vi "Grab Image from D-Link.vi"(8 "error in (no error)":errorcluster, 11 "address":string="169.254.66.10") -> (0 "error out":errorcluster, 3 "data out":string)   [LabVIEW 2012]
panel:
  out "bytes written":i32
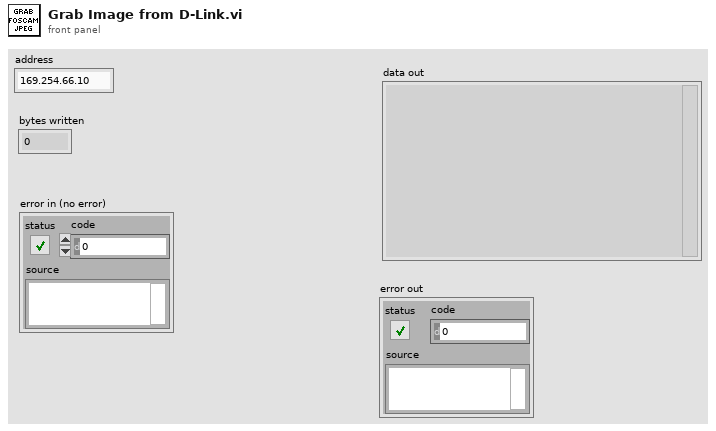
[diagram p1: front panel]
types:
  T1 = enum16{"Standard", "Buffered", "CRLF", "Immediate"}
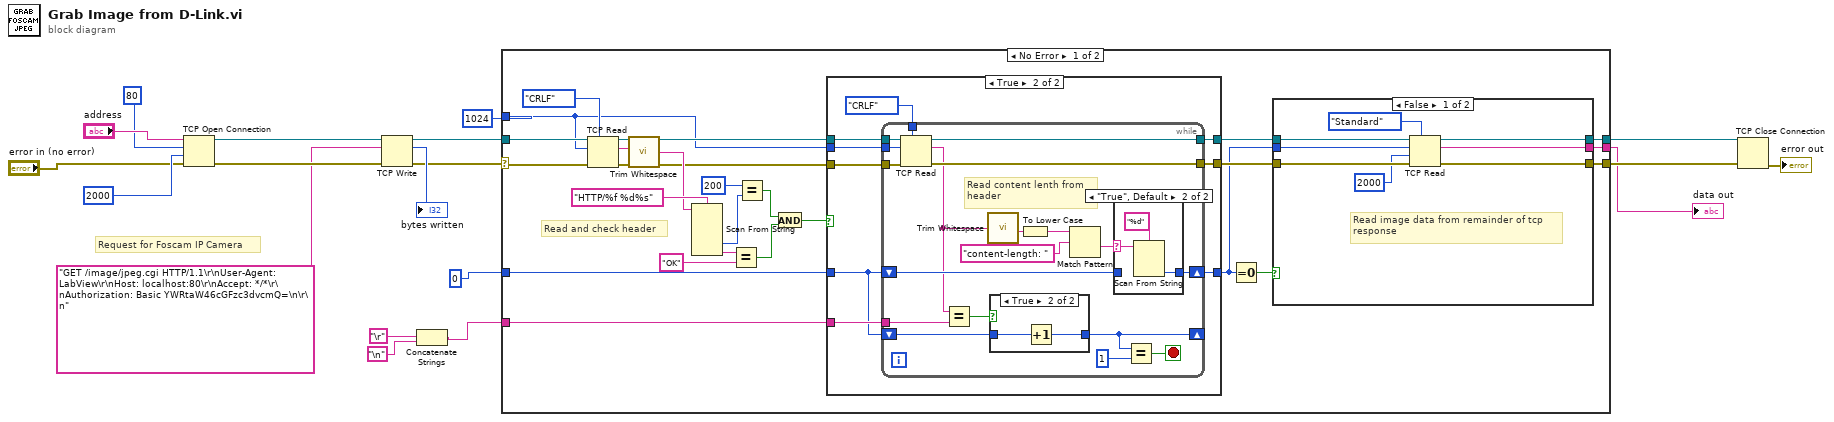
[diagram p0: block diagram]
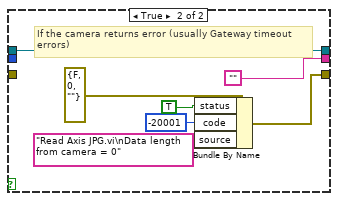
[diagram p5: hidden frame]
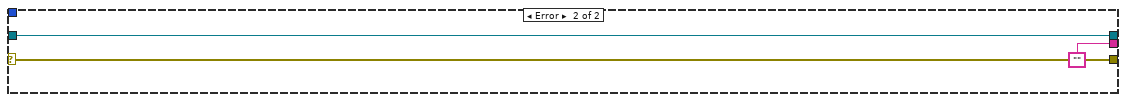
[diagram p6: hidden frame]
diagram:
  # "Request for Foscam IP Camera"
  n1 = TCP Open Connection(address="address", remote port or service name=u16 80, timeout ms (60000)=2000, error in (no error)="error in (no error)") -> (connection ID=w17:refnum<k5>, error out=w15:errorcluster)  [unwired: 1 in]
  n2 = TCP Write(connection ID=w17, data in="GET /image/jpeg.cgi HTTP/1.1\r\nUser-Agent: LabView\r\nHost: localhost:80\r\nAccept: */*\r\nAuthorization: Basic YWRtaW46cGFzc3dvcmQ=\n\r\n", error in (no error)=w15) -> (connection ID out=w11:refnum<k5>, bytes written=→"bytes written":i32, error out=w10:errorcluster)  [unwired: 1 in]
  n3 = Concatenate Strings("\r", "\n") -> (w5:string)
  n4 = case shown="No Error" w10 {
    selector: w10 -> [w22 w99]
    tunnel: [w39 w99] -> w7
    tunnel: w11 -> [w24 w97]
    tunnel: [w38 ""] -> w2
    tunnel: w5 -> [w37 _]
    tunnel: 0 -> [w36 _]
    tunnel: 1024 ("bytes to read") -> [w23 _]
    tunnel: [w35 w97] -> w8
    frame No Error {
      # "Read and check header"
      n5 = TCP Read(connection ID=w24, bytes to read=w23, error in (no error)=w22, 7:T1."CRLF" ("mode (standard)")) -> (data out=w25:string, error out=w21:errorcluster)  [unwired: 1 in, 1 out]
      n6 = call <vilib>:"Trim Whitespace.vi"("string"=w25) -> ("trimmed string"=w27:string)  [unwired: 1 in]
      n7 = Scan From String(format string="HTTP/%f %d%s", input string=w27) -> (output 2=w29:i32, output 3=w31:string)  [unwired: 6 in, 3 out]
      n8 = Equal?(x=w31, y="OK" ("format string")) -> (x = y?=w33:bool)
      n9 = Equal?(x=200, y=w29) -> (x = y?=w34:bool)
      n10 = And(x=w34, y=w33) -> (x .and. y?=w20:bool)
      n11 = case shown="True" w20 {
        tunnel: [w46 w55] -> w42
        tunnel: [w44 w54] -> w41
        tunnel: [w45 w53] -> w40
        tunnel: w37 -> [_ w52]
        tunnel: w36 -> [w44 w51]
        tunnel: w24 -> [w45 w49]
        tunnel: w23 -> [_ w48]
        tunnel: w21 -> [w46 w47]
        frame False {
        }
        frame True {
          n12 = while {
            tunnel: w49 -> [w74]
            tunnel: [w73] -> w53
            tunnel: [w72] -> w55
            shift-right: [w68] -> w54
            shift-left: w51 -> [w67]
            shift-right: [w63] -> _
            shift-left: w51 -> [w65]
            tunnel: w52 -> [w60]
            tunnel: w48 -> [w59]
            tunnel: T1."CRLF" ("mode (standard)") -> [w58]
            tunnel: w47 -> [w57]
            stop <- w64 stop-if-true
            # "Read content lenth from\nheader"
            n13 = TCP Read(connection ID=w74, bytes to read=w59, error in (no error)=w57, 7:w58) -> (connection ID out=w73:refnum<k5>, data out=w61:string, error out=w72:errorcluster)  [unwired: 1 in]
            n14 = Equal?(x=w61, y=w60) -> (x = y?=w66:bool)
            n15 = call <vilib>:"Trim Whitespace.vi"("string"=w61) -> ("trimmed string"=w70:string)  [unwired: 1 in]
            n16 = case shown="True" w66 {
              tunnel: w65 -> [w75 w77]
              tunnel: [w75 w76] -> w63
              frame False {
              }
              frame True {
                n17 = Increment(x=w77) -> (x+1=w76:i32)
              }
            }
            n18 = To Lower Case(string=w70) -> (all lower case string=w56:string)
            n19 = Match Pattern(string=w56, regular expression="content-length: ") -> (after substring=w69:string)  [unwired: 1 in, 3 out]
            n20 = case shown="\"True\", Default" w69 {
              selector: w69 -> [_ w80]
              tunnel: [w78 w81] -> w68
              tunnel: w67 -> [w78 _]
              frame "" {
              }
              frame "True", Default {
                n21 = Scan From String(format string="%d", input string=w80) -> (output 1=w81:i32)  [unwired: 3 in, 3 out]
              }
            }
            n22 = Equal?(x=w63, y=1) -> (x = y?=w64:bool)
          }
        }
      }
      n23 = Equal To 0?(x=w41) -> (x = 0?=w43:bool)
      n24 = case shown="False" w43 {
        tunnel: w40 -> [w89 w90]
        tunnel: w42 -> [w88 _]
        tunnel: [w87 w96] -> w39
        tunnel: [w83 ""] -> w38
        tunnel: w41 -> [w84 _]
        tunnel: [w82 w90] -> w35
        frame False {
          # "Read image data from remainder of tcp\nresponse"
          n25 = TCP Read(connection ID=w89, bytes to read=w84, error in (no error)=w88, 7:T1."Standard" ("mode (standard)"), 9:2000 ("timeout ms (25000)")) -> (connection ID out=w82:refnum<k5>, data out=w83:string, error out=w87:errorcluster)
        }
        frame True {
          # "If the camera returns error (usually Gateway timeout\nerrors)"
          n26 = Bundle By Name(cluster=errorcluster {"status"=FALSE, "code"=0, "source"=""} ("error in"), "status"=TRUE, "code"=-20001, "source"="Read Axis JPG.vi\nData length from camera = 0") -> (w96:errorcluster)
        }
      }
    }
    frame Error {
    }
  }
  "data out" <- w2
  n27 = TCP Close Connection(connection ID=w8, error in (no error)=w7) -> (error out=→"error out":errorcluster)  [unwired: 1 in, 1 out]
